vi "Newton Root Finding (DBL).vi"(10 "root candidate":dbl, 11 "P(x)":dbl[](array[numeric])) -> (3 "root out":dbl)   [LabVIEW 2017, in "NI_AALPro.lvlib"]
uses:
  NI_AALPro.lvlib
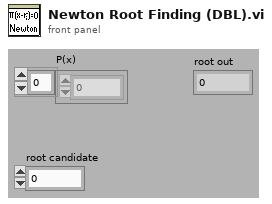
[diagram p1: front panel]
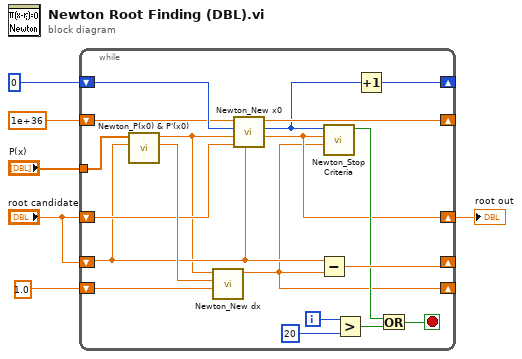
[diagram p0: block diagram]
diagram:
  n1 = while {
    shift-right: [w14] -> _
    shift-left: 1e+36 -> [w12]
    shift-right: [w23] -> _
    shift-left: "root candidate" -> [w10]
    tunnel: "P(x)" -> [w25]
    shift-right: [w15] -> w1
    shift-left: "root candidate" -> [w11]
    shift-right: [w24] -> _
    shift-left: 0 -> [w13]
    shift-right: [w9] -> _
    shift-left: 1.0 -> [w17]
    i -> [w22]
    stop <- w19 stop-if-true
    n2 = call "Newton_P(x0) & P'(x0).vi"("x0"=w10, "P(x)"=w25) -> ("P'(x0)"=w18:dbl, "P(x0)"=w7:dbl)  [unwired: 8 in]
    n3 = call "Newton_New dx.vi"("dx in"=w17, "P'(x0)"=w18, "P(x0)"=w7) -> ("dx out"=w9:dbl)  [unwired: 8 in]
    n4 = call "Newton_New x0.vi"("new x0"=w10, "x0 in"=w11, "new P(x0)"=w7, "noise in"=w13, "|P(x0)| in"=w12) -> ("x0 out"=w15:dbl, "noise out"=w8:i32, "|P(x0)| out"=w14:dbl)  [unwired: 4 in]
    n5 = Subtract(x=w10, y=w9) -> (x-y=w23:dbl)
    n6 = call "Newton_Stop Criteria.vi"("dx"=w9, "x0"=w15, "noise"=w8) -> ("stop if true"=w16:bool)  [unwired: 8 in]
    n7 = Greater?(x=w22, y=20) -> (0:w20:bool)
    n8 = Increment(x=w8) -> (x+1=w24:i32)
    n9 = Or(x=w16, y=w20) -> (x .or. y?=w19:bool)
  }
  "root out" <- w1
